vi "GLB_Fsave.vi"() -> ()   [LabVIEW 2014, in "PLS Acquisition.lvlib"]
uses:
  PLS Acquisition.lvlib
panel:
  in  "Fsave":cluster{"L1":i32, "L2":i32, "L3":i32, "L4":i32}={"L1"=10, "L2"=10, "L3"=10, "L4"=10} {"L4" items=["1 kHz"=10, "100 Hz"=100, "10 Hz"=1000, "1 Hz"=10000, "1 pt / 1 min"=600000, "1 pt / 10 min"=6000000]; "L3" items=["1 kHz"=10, "100 Hz"=100, "10 Hz"=1000, "1 Hz"=10000, "1 pt / 1 min"=600000, "1 pt / 10 min"=6000000]; "L2" items=["1 kHz"=10, "100 Hz"=100, "10 Hz"=1000, "1 Hz"=10000, "1 pt / 1 min"=600000, "1 pt / 10 min"=6000000]; "L1" items=["1 kHz"=10, "100 Hz"=100, "10 Hz"=1000, "1 Hz"=10000, "1 pt / 1 min"=600000, "1 pt / 10 min"=6000000]}
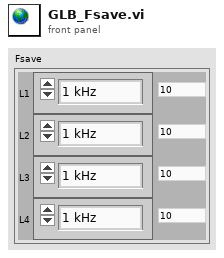
[diagram p1: front panel]
diagram:
